vi "Report Write Preset Data.vi"(8 "error in (no error)":errorcluster, 10 "report in":refnum<class "NI_report.lvclass">, 11 "Hardware Resources in":T1={"Test Setting"={"Test_Num"=0, "Test_ID"=0, "Proc_ID"=0, "Max Force"=0.0, "User"="", "SN"="", "Date"=""}, "Measurements"=[[""]], "LOG REF"=refnum, "Report Template"=path "", "Save Report path"=path "", "Data File Path"=path "", "Popup Dialog"=FALSE}) -> (0 "error out":errorcluster, 2 "report out":refnum<class "NI_report.lvclass">, 3 "Hardware Resources out":T1)   [LabVIEW 2020, in "Report.lvlib"]
doc: "Perform the acquisition. Replace the contents of this diagram with calls to acquisition hardware."
uses:
  Report.lvlib
  <vilib>/Utility/NIReport.llb/NI_report.lvclass
  <vilib>/addons/_office/_exclsub.llb/font.ctl
  <vilib>/addons/_office/NI_ReportGenerationToolkit.lvlib
  <vilib>/Utility/NIReport.llb/Word/NI_Word.lvclass
  <vilib>/Utility/NIReport.llb/Append Text Table to Report (wrap).vi
  REP Configuration.ctl
  Test Setting.ctl
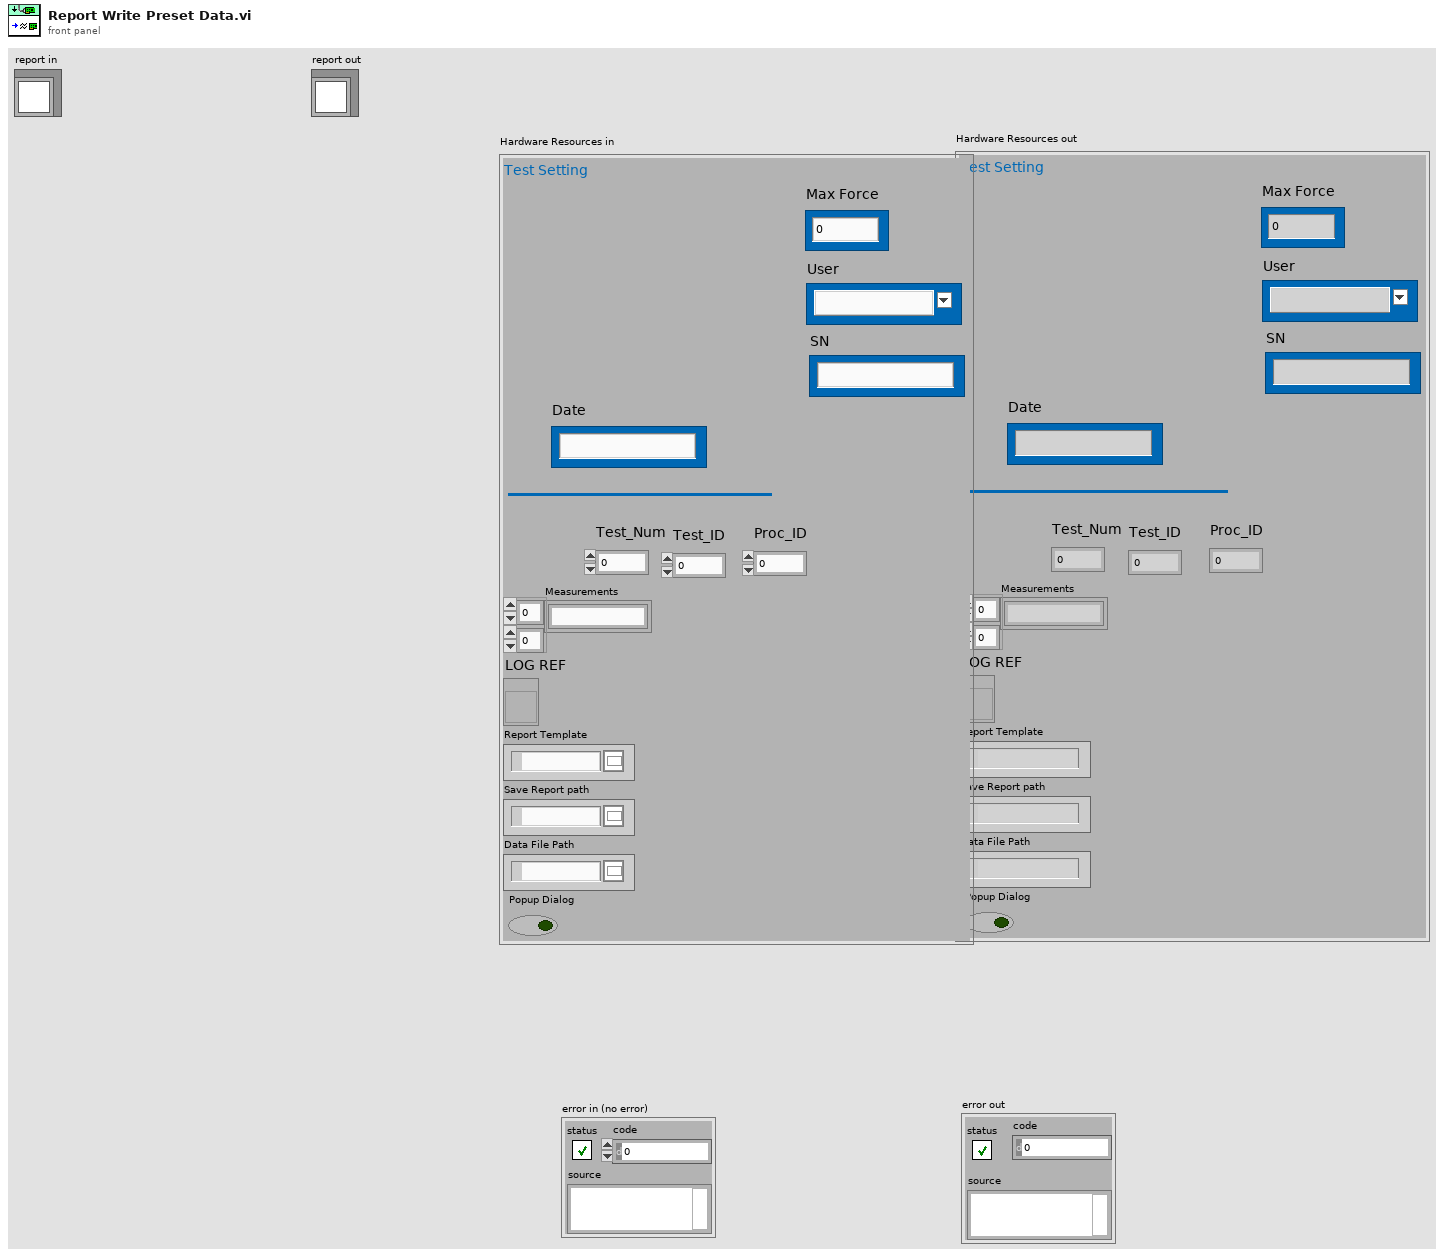
[diagram p1: front panel]
types:
  T1 = typedef "Report.lvlib/REP Configuration.ctl" = cluster{"Test Setting":T2, "Measurements":string[][], "LOG REF":refnum<vi>, "Report Template":path, "Save Report path":path, "Data File Path":path, "Popup Dialog":bool}
  T2 = typedef "Report.lvlib/Test Setting.ctl" = cluster{"Test_Num":i32, "Test_ID":i32, "Proc_ID":i32, "Max Force":dbl, "User":string, "SN":string, "Date":string}
  T3 = cluster{"position (excel)":cluster{"row":i32, "column":i32}, "name (excel)":string, "bookmark (word)":string}
  T4 = typedef "NI_ReportGenerationToolkit.lvlib/font.ctl" = cluster{"font name":string, "font size":dbl, "bold":u16, "italic":u16, "underline":u16, "strike through":u16, "font color":u32}
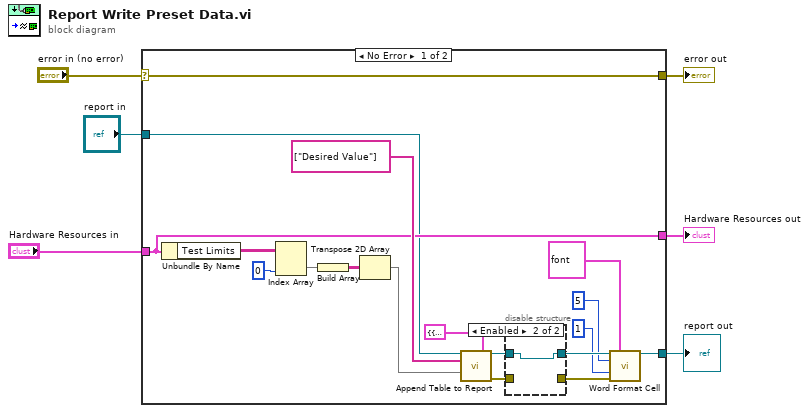
[diagram p0: block diagram]
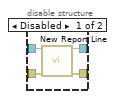
[diagram p2: hidden frame]
diagram:
  n1 = case shown="No Error" "error in (no error)" {
    selector: "error in (no error)" -> [w24 w31]
    tunnel: [w24 w31] -> w5
    tunnel: "Hardware Resources in" -> [w15 w32]
    tunnel: [w15 w32] -> w3
    tunnel: "report in" -> [w13 w30]
    tunnel: [w14 w30] -> w1
    frame No Error {
      n2 = Unbundle By Name(w15) -> ("Test Limits"=w11:string[][])
      n3 = Index Array(array=w11, index (col)=0 ("disabled index (col)")) -> (element=w9:string[])  [unwired: 1 in]
      n4 = Build Array(w9) -> (w8:string[][])
      n5 = Transpose 2D Array(2D array=w8) -> (transposed array=w7:string[][])
      n6 = call-poly <vilib>:"Append Table to Report.vi"("report in"=w13, "MS Office parameters"=T3 {"position (excel)"={"row"=0, "column"=0}, "name (excel)"="", "bookmark (word)"="Preset"}, "column headers"=string[] ["Desired Value"], "text data"=w7) -> ("report out"=w23:refnum<class "NI_report.lvclass">, "error out"=w22:errorcluster)  [unwired: 8 in, 2 out]
      n7 = disable-structure shown="Enabled" {
        disable-tunnel: w23 -> [w28 w29]
        disable-tunnel: w22 -> [w27 _]
        disable-tunnel: [w26 w29] -> w21
        disable-tunnel: [w25 _] -> w20
        frame Disabled {
          n8 = call-dynamic "New Report Line.vi"("report in"=w28, "error in (no error)"=w27) -> ("report out"=w26:refnum<class "NI_report.lvclass">, "error out"=w25:errorcluster)  [unwired: 12 in]
        }
        frame Enabled {
        }
      }
      n9 = call <vilib>:"Word Format Cell.vi"("report in"=w21, "font"=T4 {"font name"="Arial", "font size"=11.0, "bold"=2, "italic"=2, "underline"=2, "strike through"=2, "font color"=16777216}, "autoformat (-1: none)"=5, "table index (-1)"=i16 1, "error in (no error)"=w20) -> ("report out"=w14:refnum<class "NI_report.lvclass">)  [unwired: 9 in, 1 out]
    }
    frame Error {
    }
  }
  "Hardware Resources out" <- w3
  "error out" <- w5
  "report out" <- w1
